vi "Controllers.vi"() -> ()   [LabVIEW 2020]
uses:
  Classes/Controller/Controllers.ctl
  Classes/Controller/I-O/I-O.lvclass
  Classes/Controller/Dispenser/Dispenser.lvclass
  C:/Program Files (x86)/Aerotech/A3200/LabVIEW/2010/Bin/Aerotech.A3200.dll
  Program Files (x86)/Aerotech/A3200/LabVIEW/2010/Bin/Aerotech.A3200.dll
  Classes/Controller/Controller.lvclass
panel:
  in  "Cluster":T1
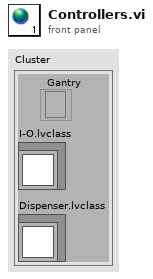
[diagram p1: front panel]
types:
  T1 = typedef "Controller.lvclass/Controllers.ctl" = cluster{"I-O.lvclass":refnum<class "I-O.lvclass">, "Dispenser.lvclass":refnum<class "Dispenser.lvclass">, "Gantry":refnum<k24>}
diagram:
